vi "GetRows.vi"(4 "error in (no error)":errorcluster, 7 "Matching Nodes":refnum<k20>[](array[refnum])) -> (0 "error out":errorcluster)   [LabVIEW 2014, in "Spreadsheet.lvclass"]
uses:
  Spreadsheet.lvclass
  XML.lvlib
  <resource>/objmgr/DOMUserDefRef.rc
panel:
  out "Cell Info":string[][](array[string])
  out "Table Data":string[][](array[string])
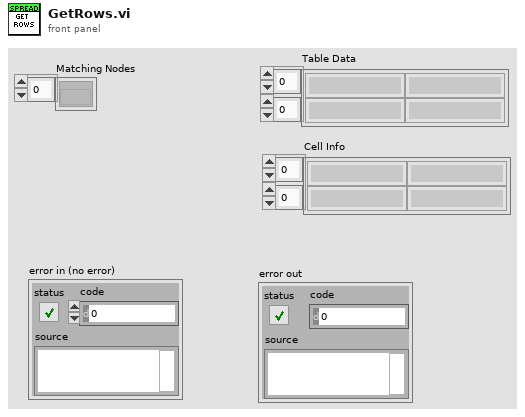
[diagram p1: front panel]
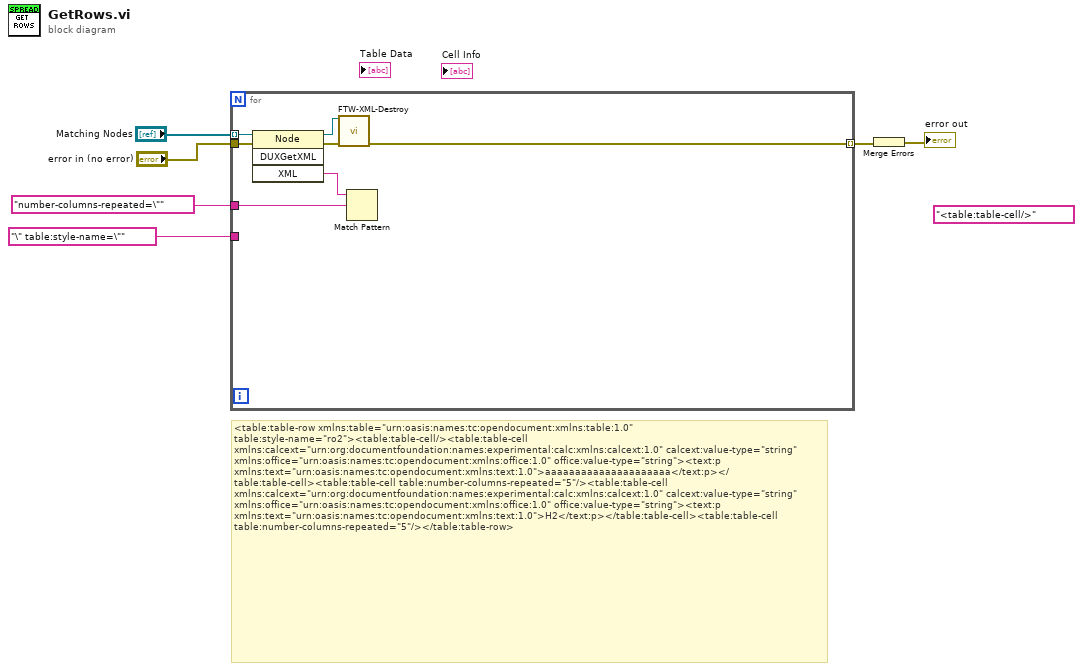
[diagram p0: block diagram]
diagram:
  (unwired) "<table:table-cell/>"
  # "<table:table-row xmlns:table=\"urn:oasis:names:tc:opendocument:xmlns:table:1.0\" table:style-name=\"ro2\"><table:table-cell/><table:table-cell xmlns:calcext=\"urn:org:documentfoundation:names:experimental:calc:xmlns:calcext:1.0\" calcext:value-type=\"string\" xmlns:office=\"urn:oasis:names:tc:opendocument:xmlns:office:1.0\" office:value-type=\"string\"><text:p xmlns:text=\"urn:oasis:names:tc:opendocument:xmlns:text:1.0\">aaaaaaaaaaaaaaaaaaaaa</text:p></table:table-cell><table:table-cell table:number-columns-repeated=\"5\"/><table:table-cell xmlns:calcext=\"urn:org:documentfoundation:names:experimental:calc:xmlns:calcext:1.0\" calcext:value-type=\"string\" xmlns:office=\"urn:oasis:names:tc:opendocument:xmlns:office:1.0\" office:value-type=\"string\"><text:p xmlns:text=\"urn:oasis:names:tc:opendocument:xmlns:text:1.0\">H2</text:p></table:table-cell><table:table-cell table:number-columns-repeated=\"5\"/></table:table-row>"
  n1 = for {
    tunnel: "Matching Nodes" -> [w13] mode=indexing
    tunnel: "error in (no error)" -> [w12]
    tunnel: "number-columns-repeated=\"" -> [w8]
    tunnel: "\" table:style-name=\"" -> [_]
    tunnel: [w7] -> w1 mode=indexing
    n2 = invoke class="Node" method="DUXGetXML"(reference=w13, error in=w12) -> (reference out=w10:refnum<k20>, error out=w11:errorcluster, "XML"=w9:string)  [unwired: 2 in, 1 out]
    n3 = call "FTW-XML-Destroy.vi"("XML Node"=w10, "error in"=w11) -> ("error out"=w7:errorcluster)  [unwired: 13 in]
    n4 = Match Pattern(string=w9, regular expression=w8) -> ()  [unwired: 1 in, 4 out]
  }
  n5 = Merge Errors(w1) -> (→"error out":errorcluster)
